vi "7HP.vi"() -> (0 "DAQ Error":errorcluster)   [LabVIEW 2021]
doc: "Use this plug-in with the Nathan 7609 data acquisition system"
uses:
  Analysis/7 Hole Probe pressures to UVW/7HP_Global.vi
  Globals/Meas_global.vi
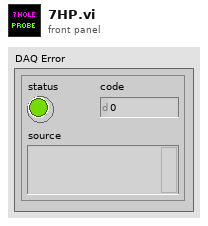
[diagram p1: front panel]
types:
  T1 = typedef "Device ID port info.ctl" = cluster{"Ch No":i16[], "Req Sampling Rate":dbl[], "Port":string, "Index":i32[]}
  T2 = typedef "Setup.ctl" = enum16{"Run Program", "Show Setup", "Save Current Setup", "Setup Front Panel"}
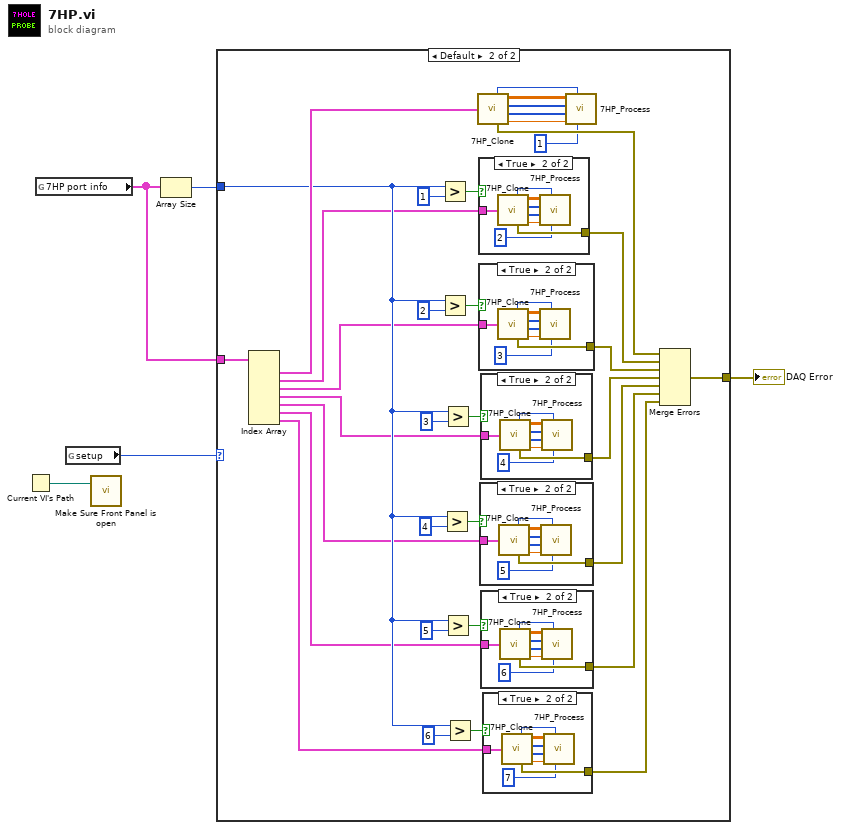
[diagram p0: block diagram]
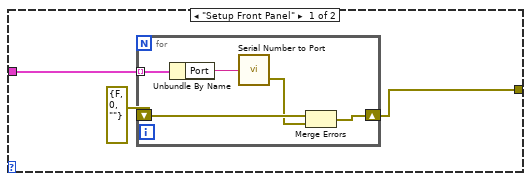
[diagram p2: hidden frame]
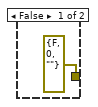
[diagram p3: hidden frame]
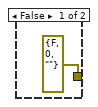
[diagram p4: hidden frame]
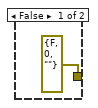
[diagram p5: hidden frame]
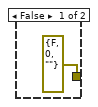
[diagram p6: hidden frame]
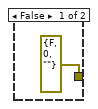
[diagram p7: hidden frame]
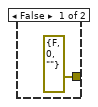
[diagram p8: hidden frame]
diagram:
  n1 = Current VI's Path() -> (path=w1:path)
  n2 = global read "7HP_Global.vi" "7HP port info"() -> (w2:T1[])
  n3 = global read "Meas_global.vi" "setup"() -> (w3:T2)
  n4 = call "Make Sure Front Panel is open.vi"("path"=w1) -> ()
  n5 = Array Size(array=w2) -> (size(s)=w5:i32)
  n6 = case shown="Default" w3 {
    tunnel: w2 -> [w8 w48]
    tunnel: w5 -> [_ w30]
    tunnel: [w6 w16] -> w4
    frame "Setup Front Panel" {
      n7 = for {
        tunnel: w8 -> [w13] mode=indexing
        shift-right: [w9] -> w6
        shift-left: errorcluster {"status"=FALSE, "code"=0, "source"=""} ("error IO") -> [w11]
        n8 = Unbundle By Name(w13) -> ("Port"=w12:string)
        n9 = call "Serial Number to Port.vi"("Port In"=w12) -> ("error out"=w10:errorcluster)  [unwired: 1 out]
        n10 = Merge Errors(w11, w10) -> (w9:errorcluster)
      }
    }
    frame Default {
      n11 = Index Array(array=w48) -> (element #1=w43:T1, element #2=w29:T1, element #3=w28:T1, element #4=w27:T1, element #5=w26:T1, element #6=w25:T1, element #7=w24:T1)  [unwired: 7 in]
      n12 = Greater?(x=w30, y=1) -> (0:w41:bool)
      n13 = Greater?(x=w30, y=2) -> (0:w40:bool)
      n14 = Greater?(x=w30, y=4) -> (0:w36:bool)
      n15 = Greater?(x=w30, y=3) -> (0:w37:bool)
      n16 = Greater?(x=w30, y=5) -> (0:w33:bool)
      n17 = Greater?(x=w30, y=6) -> (0:w32:bool)
      n18 = call "7HP_Clone.vi"("Single 7HP"=w43) -> ("Serial number"=w15:u32, "DAQ Error"=w22:errorcluster, "All samples out"=w44:sgl[][], "Ch No"=w45:i16[], "Index"=w46:i32[], "Sampling Rate Hz"=w47:dbl)
      n19 = case shown="True" w41 {
        tunnel: w29 -> [_ w98]
        tunnel: [errorcluster {"status"=FALSE, "code"=0, "source"=""} ("DAQ Error") w97] -> w23
        frame False {
        }
        frame True {
          n20 = call "7HP_Clone.vi"("Single 7HP"=w98) -> ("Serial number"=w95:u32, "DAQ Error"=w97:errorcluster, "All samples out"=w102:sgl[][], "Ch No"=w101:i16[], "Index"=w100:i32[], "Sampling Rate Hz"=w99:dbl)
          n21 = call "7HP_Process.vi"("All samples in"=w102, "Serial number"=w95, "7HP Ch No"=w101, "Analysis info Index"=w100, "Probe Number"=2, "Sampling Rate"=w99) -> ()  [unwired: 3 in]
        }
      }
      n22 = case shown="True" w40 {
        tunnel: w28 -> [_ w89]
        tunnel: [errorcluster {"status"=FALSE, "code"=0, "source"=""} ("DAQ Error") w88] -> w21
        frame False {
        }
        frame True {
          n23 = call "7HP_Clone.vi"("Single 7HP"=w89) -> ("Serial number"=w86:u32, "DAQ Error"=w88:errorcluster, "All samples out"=w93:sgl[][], "Ch No"=w92:i16[], "Index"=w91:i32[], "Sampling Rate Hz"=w90:dbl)
          n24 = call "7HP_Process.vi"("All samples in"=w93, "Serial number"=w86, "7HP Ch No"=w92, "Analysis info Index"=w91, "Probe Number"=3, "Sampling Rate"=w90) -> ()  [unwired: 3 in]
        }
      }
      n25 = case shown="True" w36 {
        tunnel: w26 -> [_ w71]
        tunnel: [errorcluster {"status"=FALSE, "code"=0, "source"=""} ("DAQ Error") w70] -> w19
        frame False {
        }
        frame True {
          n26 = call "7HP_Clone.vi"("Single 7HP"=w71) -> ("Serial number"=w68:u32, "DAQ Error"=w70:errorcluster, "All samples out"=w75:sgl[][], "Ch No"=w74:i16[], "Index"=w73:i32[], "Sampling Rate Hz"=w72:dbl)
          n27 = call "7HP_Process.vi"("All samples in"=w75, "Serial number"=w68, "7HP Ch No"=w74, "Analysis info Index"=w73, "Probe Number"=5, "Sampling Rate"=w72) -> ()  [unwired: 3 in]
        }
      }
      n28 = case shown="True" w37 {
        tunnel: w27 -> [_ w80]
        tunnel: [errorcluster {"status"=FALSE, "code"=0, "source"=""} ("DAQ Error") w79] -> w20
        frame False {
        }
        frame True {
          n29 = call "7HP_Clone.vi"("Single 7HP"=w80) -> ("Serial number"=w77:u32, "DAQ Error"=w79:errorcluster, "All samples out"=w84:sgl[][], "Ch No"=w83:i16[], "Index"=w82:i32[], "Sampling Rate Hz"=w81:dbl)
          n30 = call "7HP_Process.vi"("All samples in"=w84, "Serial number"=w77, "7HP Ch No"=w83, "Analysis info Index"=w82, "Probe Number"=4, "Sampling Rate"=w81) -> ()  [unwired: 3 in]
        }
      }
      n31 = case shown="True" w33 {
        tunnel: w25 -> [_ w62]
        tunnel: [errorcluster {"status"=FALSE, "code"=0, "source"=""} ("DAQ Error") w61] -> w18
        frame False {
        }
        frame True {
          n32 = call "7HP_Clone.vi"("Single 7HP"=w62) -> ("Serial number"=w59:u32, "DAQ Error"=w61:errorcluster, "All samples out"=w66:sgl[][], "Ch No"=w65:i16[], "Index"=w64:i32[], "Sampling Rate Hz"=w63:dbl)
          n33 = call "7HP_Process.vi"("All samples in"=w66, "Serial number"=w59, "7HP Ch No"=w65, "Analysis info Index"=w64, "Probe Number"=6, "Sampling Rate"=w63) -> ()  [unwired: 3 in]
        }
      }
      n34 = case shown="True" w32 {
        tunnel: w24 -> [_ w53]
        tunnel: [errorcluster {"status"=FALSE, "code"=0, "source"=""} ("DAQ Error") w52] -> w17
        frame False {
        }
        frame True {
          n35 = call "7HP_Clone.vi"("Single 7HP"=w53) -> ("Serial number"=w50:u32, "DAQ Error"=w52:errorcluster, "All samples out"=w57:sgl[][], "Ch No"=w56:i16[], "Index"=w55:i32[], "Sampling Rate Hz"=w54:dbl)
          n36 = call "7HP_Process.vi"("All samples in"=w57, "Serial number"=w50, "7HP Ch No"=w56, "Analysis info Index"=w55, "Probe Number"=7, "Sampling Rate"=w54) -> ()  [unwired: 3 in]
        }
      }
      n37 = call "7HP_Process.vi"("All samples in"=w44, "Serial number"=w15, "7HP Ch No"=w45, "Analysis info Index"=w46, "Probe Number"=1, "Sampling Rate"=w47) -> ()  [unwired: 3 in]
      n38 = Merge Errors(w22, w23, w21, w20, w19, w18, w17) -> (w16:errorcluster)
    }
  }
  "DAQ Error" <- w4
